vi "testLoopbackUDP.vi"(8 "error in (no error)":errorcluster, 11 "TestCase in":refnum<class "DSF CD System Tests.lvclass">) -> (0 "error out":errorcluster, 3 "TestCase out":refnum<class "DSF CD System Tests.lvclass">)   [LabVIEW 2017, in "DSF CD System Tests.lvclass"]
uses:
  DSF CD System Tests.lvclass
  C:/Git/niveristand-custom-device-testing-tools/VeriStandTestCase/VeriStandTestCase.lvclass
  b55b5565-dc34-4e51-bcfa-5a6cba25043e.vi
  df0c3853-f0b6-44a9-ad36-32614d313efc.vi
  <vilib>/NI Veristand/Execution/Workspace/NI VeriStand - Set Single Channel Value.vi
  <vilib>/NI Veristand/Execution/Workspace/NI VeriStand - Get Single Channel Value.vi
  <vilib>/addons/_JKI Toolkits/VI Tester/TestCase.llb/TestCase.lvclass
  <vilib>/NI VeriStand/Execution/Workspace/NI_VS Workspace ExecutionAPI.lvlib
  C:/Program Files (x86)/National Instruments/LabVIEW 2017/vi.lib/addons/_JKI Toolkits/VI Tester/TestCase.llb/TestCase.lvclass
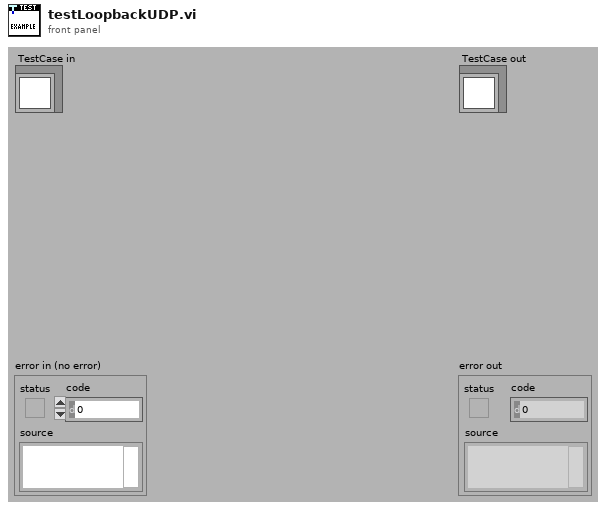
[diagram p1: front panel]
types:
  T1 = typedef "NI_VS Workspace ExecutionAPI.lvlib/WorkspaceAPI.ctl" = refnum<k24>
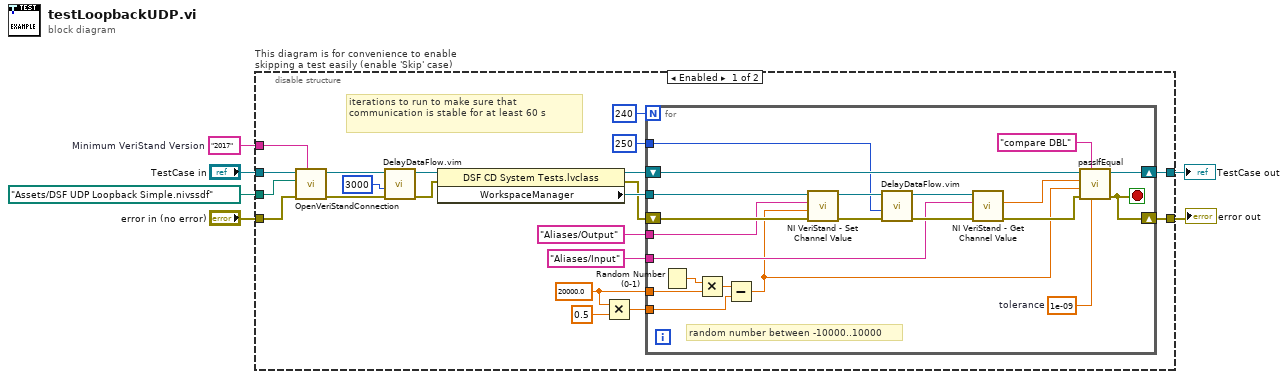
[diagram p0: block diagram]
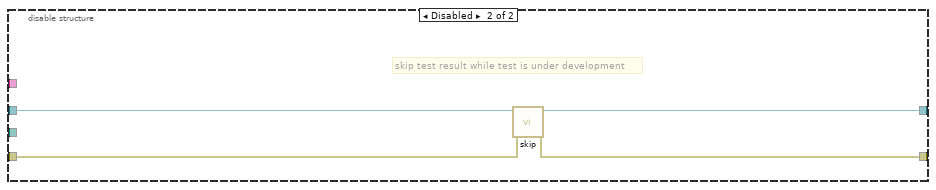
[diagram p2: hidden frame]
diagram:
  w1 = "2017"  # Minimum VeriStand Version
  n1 = disable-structure "This diagram is for convenience to enable skipping a test easily (enable 'Skip' case)" shown="Enabled" {
    disable-tunnel: "TestCase in" -> [w25 w50]
    disable-tunnel: [w18 w48] -> w3
    disable-tunnel: [w17 w49] -> w5
    disable-tunnel: "error in (no error)" -> [w26 w47]
    disable-tunnel: path "Assets/DSF UDP Loopback Simple.nivssdf" ("System Definition File") -> [w13 _]
    disable-tunnel: w1 -> [w12 _]
    frame Enabled {
      w8 = 20000.0 ("y")
      # "iterations to run to make sure that communication is stable for at least 60 s"
      n2 = call-dynamic "OpenVeriStandConnection.vi"("Minimum VeriStand Version (2016)"=w12, "error in (no error)"=w26, "System Definition File"=w13, "VeriStand Test Case in"=w25) -> ("error out"=w15:errorcluster, "VeriStand Test Case out"=w24:refnum<class "DSF CD System Tests.lvclass">)  [unwired: 5 in, 1 out]
      n3 = call "DelayDataFlow.vim"("value in"=w15, "milliseconds to wait"=u32 3000) -> ("value out"=w14:errorcluster)  [unwired: 2 in, 1 out]
      n4 = property class="DSF CD System Tests.lvclass"(reference=w24, error in=w14) -> (reference out=w19:refnum<class "DSF CD System Tests.lvclass">, error out=w22:errorcluster, "WorkspaceManager"=w23:T1)
      n5 = Multiply(x=w8, y=0.5) -> (x*y=w9:dbl)
      n6 = for {
        N: 240 -> [_]
        tunnel: w23 -> [w46]
        tunnel: "Aliases/Input" ("Channel") -> [w41]
        tunnel: "Aliases/Output" ("Channel") -> [w40]
        shift-right: [w27] -> w17
        shift-left: w22 -> [w45]
        shift-right: [w36] -> w18
        shift-left: w19 -> [w37]
        tunnel: w9 -> [w30]
        tunnel: w8 -> [w29]
        tunnel: u32 250 ("milliseconds to wait") -> [w28]
        stop <- w27 stop-if-true
        w32 = 1e-09  # tolerance
        # "random number between -10000..10000"
        n7 = Random Number (0-1)() -> (number: 0 to 1=w35:dbl)
        n8 = Multiply(x=w35, y=w29) -> (x*y=w34:dbl)
        n9 = Subtract(x=w34, y=w30) -> (x-y=w33:dbl)
        n10 = call-poly <vilib>:"NI VeriStand - Set Channel Value.vi"("error in (no error)"=w45, "Value"=w33, "Channel"=w40, "WorkspaceManager in"=w46) -> ("error out"=w44:errorcluster, "WorkspaceManager out"=w42:T1)  [unwired: 6 in]
        n11 = call "DelayDataFlow.vim"("value in"=w44, "milliseconds to wait"=w28) -> ("value out"=w43:errorcluster)  [unwired: 2 in, 1 out]
        n12 = call-poly <vilib>:"NI VeriStand - Get Channel Value.vi"("error in (no error)"=w43, "Channel"=w41, "WorkspaceManager in"=w42) -> ("error out"=w39:errorcluster, "Value"=w38:dbl)  [unwired: 6 in, 1 out]
        n13 = call-dynamic "passIfEqual.vi"("delta (optional)"=w32, "custom report message (\"\")"="compare DBL" ("custom report message (\"\")"), "error in (no error)"=w39, "y"=w33, "x"=w38, "TestCase in"=w37) -> ("error out"=w27:errorcluster, "TestCase out"=w36:refnum<class "DSF CD System Tests.lvclass">)  [unwired: 4 in]
      }
    }
    frame Disabled {
      # "skip test result while test is under development"
      n14 = call <vilib>:"skip.vi"("error in (no error)"=w47, "TestCase in"=w50) -> ("error out"=w49:errorcluster, "TestCase out"=w48:refnum<class "DSF CD System Tests.lvclass">)  [unwired: 8 in]
    }
  }
  "error out" <- w5
  "TestCase out" <- w3
